vi "Log DAQ event.vi"(8 "error in (no error)":errorcluster, 9 "BoolState":bool, 10 "IOName":string, 11 "Refnum in":refnum<k34>) -> (0 "error out":errorcluster)   [LabVIEW 2017, in "DAQ.lvclass"]
doc: "Developed by Kevin Thompson\nkevin@thompsonengineering.net\n\nCopyright 2018-2020\nThompson Engineering, LLC"
uses:
  DAQ.lvclass
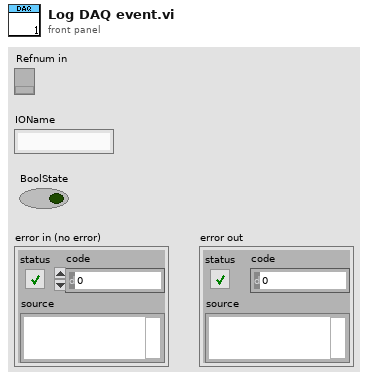
[diagram p1: front panel]
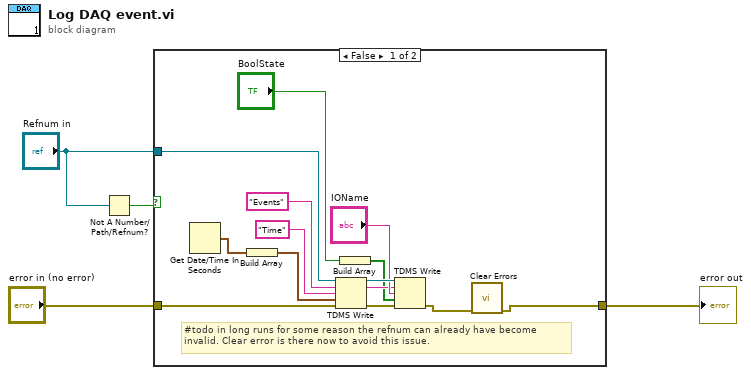
[diagram p0: block diagram]
diagram:
  n1 = Not A Number/Path/Refnum?(number/path/refnum="Refnum in") -> (NaN/Path/Refnum?=w1:bool)
  n2 = case shown="False" w1 {
    tunnel: [w5 w19] -> w4
    tunnel: "error in (no error)" -> [w17 w19]
    tunnel: "Refnum in" -> [w16 _]
    frame False {
      # "#todo in long runs for some reason the refnum can already have become\ninvalid. Clear error is there now to avoid this issue."
      n3 = Get Date/Time In Seconds() -> (seconds since 1Jan1904=w7:timestamp)
      n4 = Build Array(w7) -> (w8:timestamp[])
      n5 = TDMS Write(0:w16, 5:"Events" ("group name"), 7:"Time" ("channel name"), 9:w8, 11:w17) -> (4:w15:refnum<k34>, 6:w12:string, 15:w18:errorcluster)  [unwired: 1 in, 1 out]
      n6 = Build Array("BoolState") -> (w10:bool[])
      n7 = TDMS Write(0:w15, 5:w12, 7:"IOName", 9:w10, 11:w18) -> (15:w6:errorcluster)  [unwired: 1 in, 3 out]
      n8 = call <vilib>:"Clear Errors.vi"("error in (no error)"=w6) -> ("error out"=w5:errorcluster)  [unwired: 5 in, 1 out]
    }
    frame True {
    }
  }
  "error out" <- w4
